vi "SUB_ReadLogFile.vi"() -> (0 "error out":errorcluster, 1 "text":string)   [LabVIEW 2011]
panel:
  out "path":path
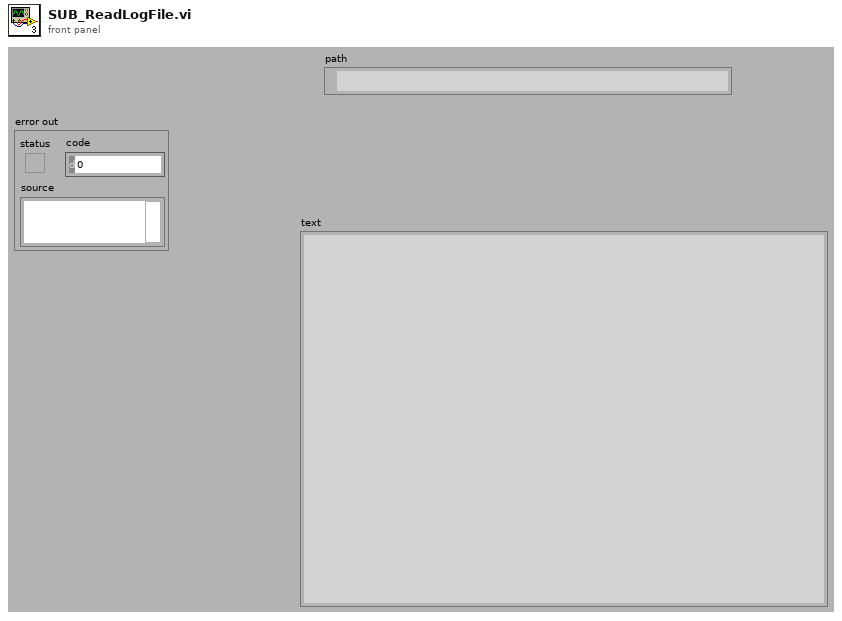
[diagram p1: front panel]
types:
  T1 = enum32{"invalid app kind", "Development System", "Run Time System", "Student Edition", "Embedded LabVIEW", "Evaluation", "Custom"}
  T2 = enum16{"open", "replace", "create", "open or create", "replace or create", "replace or create with confirmation"}
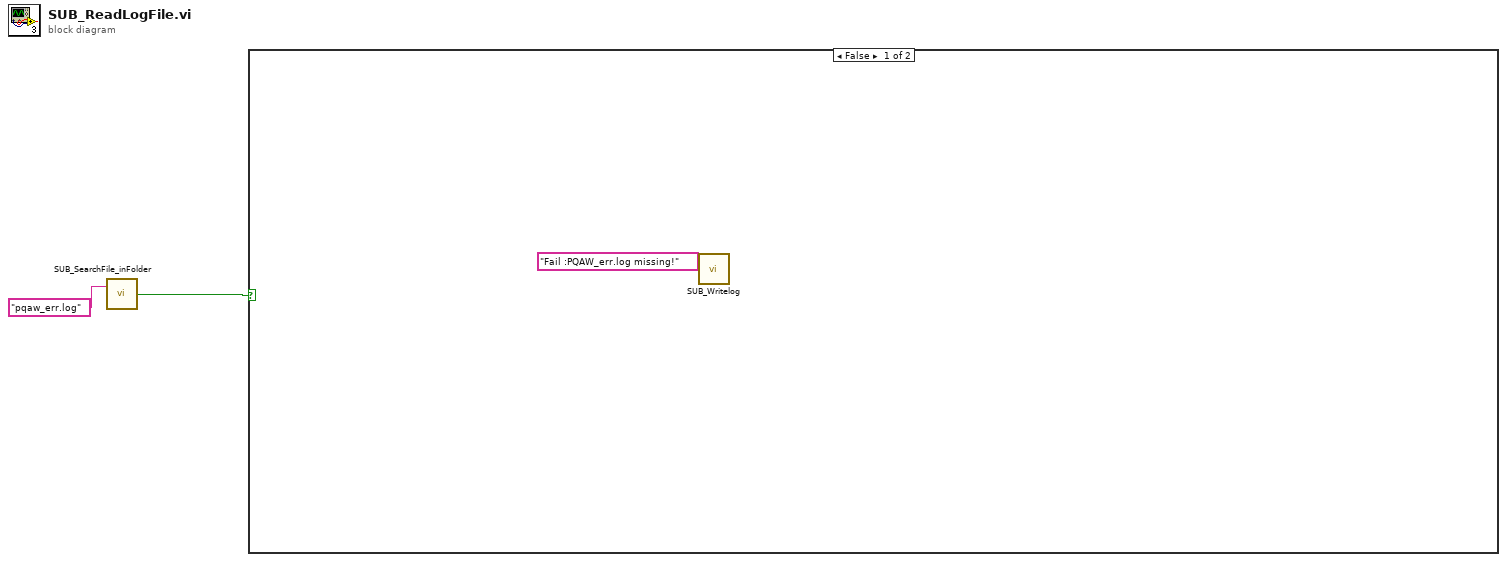
[diagram p0: block diagram]
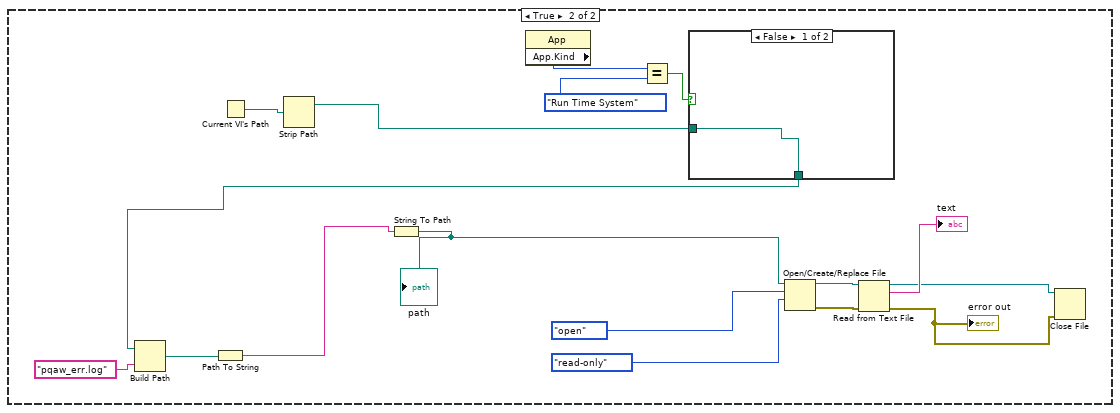
[diagram p2: hidden frame]
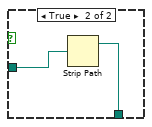
[diagram p3: hidden frame]
diagram:
  n1 = call "SUB_SearchFile_inFolder.vi"("Search Filename in Folder"="pqaw_err.log" ("string")) -> ("File Existing True/Flase"=w1:bool)  [unwired: 1 in]
  n2 = case shown="False" w1 {
    frame False {
      n3 = call "SUB_Writelog.vi"("Pass/Fail"="Fail :PQAW_err.log missing!") -> ()  [unwired: 2 in]
    }
    frame True {
      n4 = Current VI's Path() -> (path=w15:path)
      n5 = Strip Path(path=w15) -> (stripped path=w11:path)  [unwired: 1 out]
      n6 = property class="App"() -> ("App.Kind"=w14:T1)  [unwired: 2 in, 2 out]
      n7 = Equal?(x=w14, y=T1."Run Time System" ("Application:Kind")) -> (x = y?=w12:bool)
      n8 = case shown="False" w12 {
        tunnel: w11 -> [w21 w23]
        tunnel: [w21 w22] -> w5
        frame False {
        }
        frame True {
          n9 = Strip Path(path=w23) -> (stripped path=w22:path)  [unwired: 1 out]
        }
      }
      n10 = Build Path(base path=w5, name or relative path="pqaw_err.log" ("string")) -> (appended path=w7:path)
      n11 = Path To String(path=w7) -> (string=w4:string)
      n12 = String To Path(string=w4) -> (path=w10:path)
      "path" <- w10
      n13 = Open/Create/Replace File(file path (use dialog)=w10, operation (0:open)=T2."open", access (0:read/write)=enum16{"read/write", "read-only", "write-only"}."read-only") -> (refnum out=w18:refnum<file>, error out=w17:errorcluster)  [unwired: 3 in, 1 out]
      n14 = Read from Text File(file (use dialog)=w18, error in=w17) -> (refnum out=w9:refnum<file>, text=→"text":string, error out=w8:errorcluster)  [unwired: 2 in, 1 out]
      "error out" <- w8
      n15 = Close File(refnum=w9, error in=w8) -> ()  [unwired: 2 out]
    }
  }
